vi "GetRandomString.vi"(8 "error in (no error)":errorcluster, 11 "Generator in":refnum<class "Generator.lvclass">) -> (0 "error out":errorcluster, 3 "Generator out":refnum<class "Generator.lvclass">)   [LabVIEW 2021, in "Generator.lvlib" / "Generator.lvclass"]
uses:
  Generator.lvclass
  Generator.lvclass/Generator.ctl
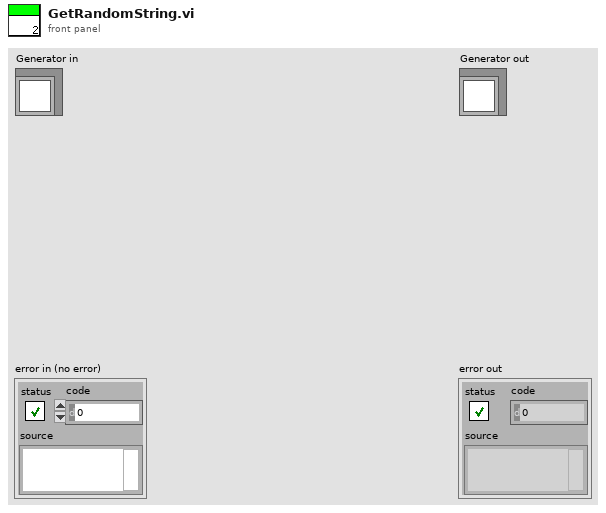
[diagram p1: front panel]
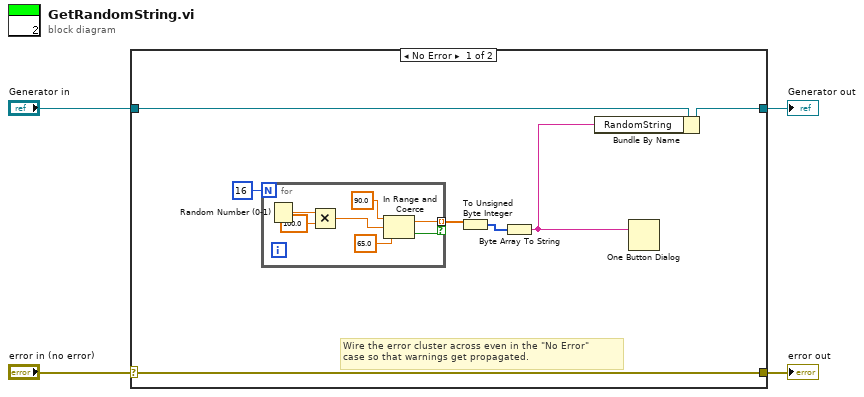
[diagram p0: block diagram]
diagram:
  n1 = case shown="No Error" "error in (no error)" {
    selector: "error in (no error)" -> [w10 w20]
    tunnel: [w10 w20] -> w3
    tunnel: [w6 w19] -> w1
    tunnel: "Generator in" -> [w11 w19]
    frame No Error {
      # "Wire the error cluster across even in the \"No Error\"\ncase so that warnings get propagated."
      n2 = for {
        N: 16 -> [_]
        tunnel: [w13] -> w8 mode=indexing if=w12
        n3 = Random Number (0-1)() -> (number: 0 to 1=w18:dbl)
        n4 = Multiply(x=w18, y=100.0) -> (x*y=w17:dbl)
        n5 = In Range and Coerce(upper limit=90.0, x=w17, lower limit=65.0) -> (coerced(x)=w13:dbl, In Range?=w12:bool)
      }
      n6 = To Unsigned Byte Integer(number=w8) -> (unsigned 8bit integer=w7:u8[])
      n7 = Byte Array To String(unsigned byte array=w7) -> (string=w5:string)
      n8 = Bundle By Name(cluster=w11, "RandomString"=w5) -> (w6:refnum<class "Generator.lvclass">)
      n9 = One Button Dialog(message=w5) -> ()  [unwired: 1 in, 1 out]
    }
    frame Error {
    }
  }
  "error out" <- w3
  "Generator out" <- w1
